vi "Autonomous.vi"() -> ()   [LabVIEW 2023]
doc: "This VI starts when autonomous period begins, and will automatically be terminated when it ends. You can carry out timed or sensor driven operations directly to I/O or to subsystems without needing to return to the caller."
uses:
  <vilib>/Rock Robotics/WPI/Utilities/WPI_GetSetVariantRefNum.vi
  Framework/Robot Global Data.vi
  <vilib>/Rock Robotics/Network Tables/NT Read String.vi
  <vilib>/Rock Robotics/Network Tables/NT Read String Array.vi
  <vilib>/Utility/file.llb/Read Delimited Spreadsheet (string).vi
panel:
  in  "Is Blue Alliance?":bool=TRUE
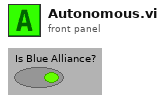
[diagram p1: front panel]
types:
  T1 = typedef "WPI_JoystickDevRef.ctl" = cluster{"Device":T2}
  T2 = typedef "WPI_JoystickDeviceEnum.ctl" = enum16{"USB 0", "USB 1", "USB 2", "USB 3", "USB 4", "USB 5"}
  T3 = typedef "Robot Velocities.ctl" = cluster{"X Velocity":dbl, "Y Velocity":dbl, "Rotational \nVelocity":dbl}
  T4 = typedef "Single Cmd Info.ctl" = cluster{"Name":string, "CPTM.DataType":variant, "All Control Values Variant":cluster{"Name":string, "Variant Data":variant}[], "icon full":T5, "icon scaled":T5, "Path":path, "Subsystem Color":u32}
  T5 = typedef "imagedata.ctl" = cluster{"image type":i32, "image depth":i32, "image":u8[], "mask":u8[], "colors":u32[], "Rectangle":cluster{"left":i16, "top":i16, "right":i16, "bottom":i16}}
  T6 = cluster{"Name":string, "vi reference":refnum<vi>, i32[], variant[]}
  T7 = cluster{dbl, "Command out":cluster{"Name":string, "vi reference":refnum<vi>, i32[], variant[]}}
  T8 = cluster{dbl, "Command out":cluster{"Name":string, "vi reference":refnum<vi>, i32[], variant[]}}[]
  T9 = cluster{"Velocities":T3[], "Positions":cluster{"x":dbl, "y":dbl, "th":dbl}[], cluster{dbl, "Command out":cluster{"Name":string, "vi reference":refnum<vi>, i32[], variant[]}}[], "Zero Velocity?":bool[]}
  T10 = typedef "CTRE_PigeonIMU_DeviceRef.ctl" = cluster{"DeviceStatus":errorcluster, "Device Number":u8, "Type":T11, "Device ID":u32, "Handle":u64, "UsageFrame":u32, "Library Path":path}
  T11 = typedef "CTRE_PigeonIMU_ConnectionType.ctl" = u32
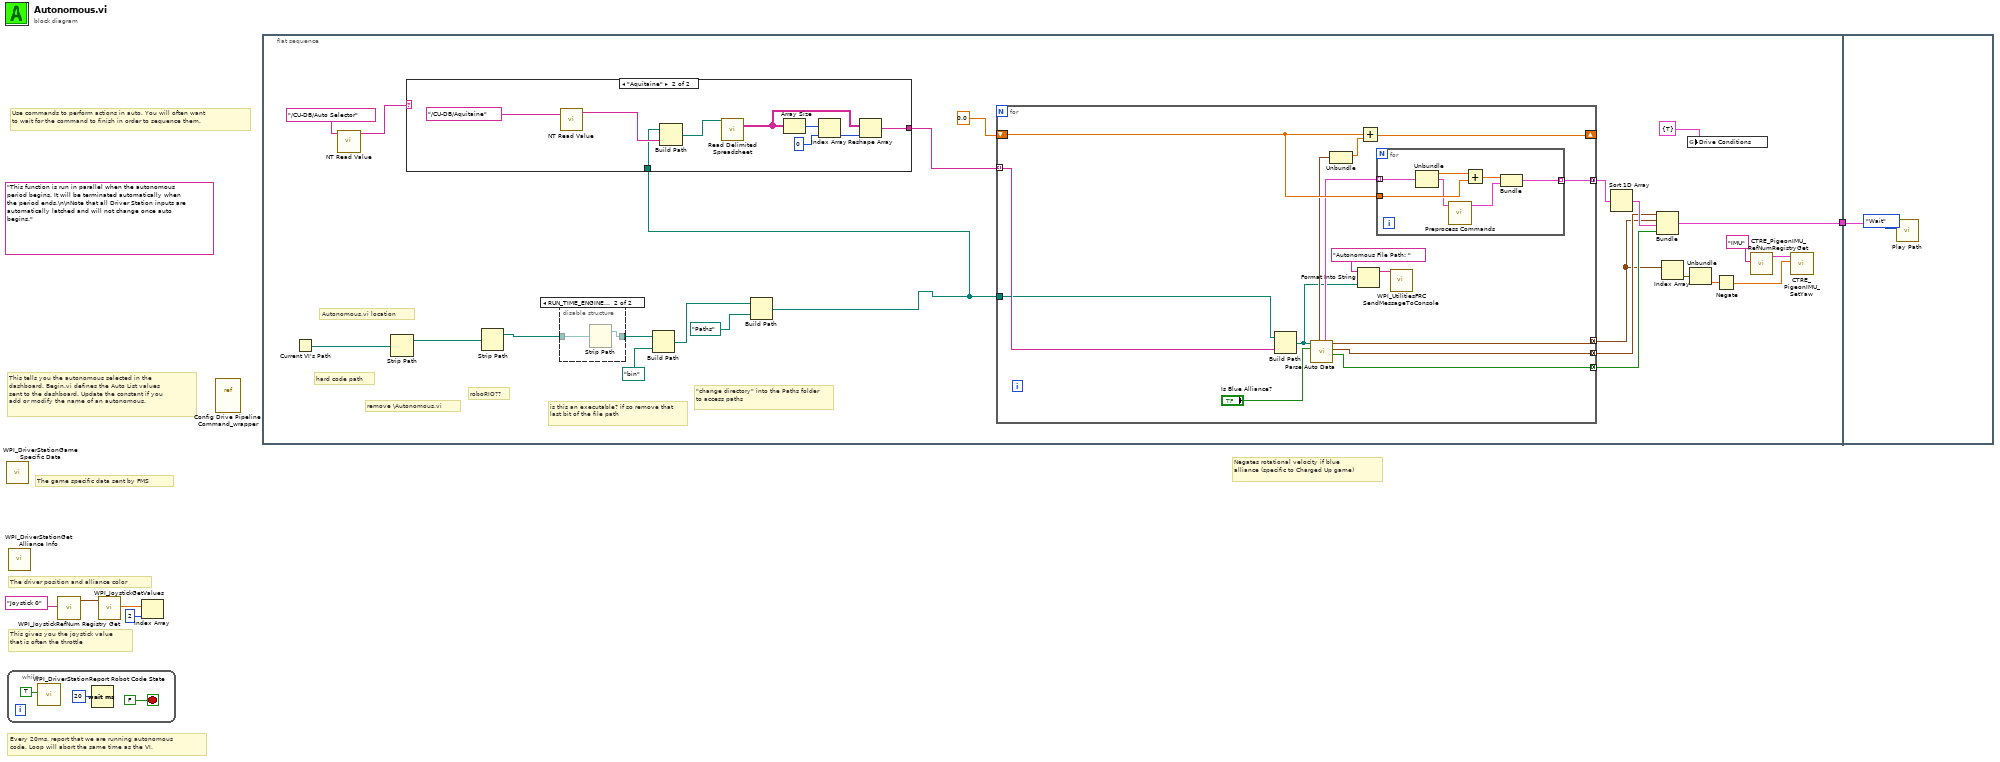
[diagram p0: block diagram]
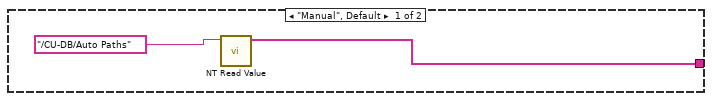
[diagram p3: hidden frame]
diagram:
  (unwired) "This function is run in parallel when the autonomous period begins. It will be terminated automatically when the period ends.\n\nNote that all Driver Station inputs are automatically latched and will not change once auto begins."
  # "Negates rotational velocity if blue alliance (specific to Charged Up game)"
  # "The game specific data sent by FMS"
  # "This tells you the autonomous selected in the \ndashboard. Begin.vi defines the Auto List values\nsent to the dashboard. Update the constant if you\nadd or modify the name of an autonomous."
  # "Every 20ms, report that we are running autonomous\ncode. Loop will abort the same time as the VI."
  # "This gives you the joystick value\nthat is often the throttle"
  # "Use commands to perform actions in auto. You will often want\nto wait for the command to finish in order to sequence them."
  # "The driver position and alliance color"
  n1 = call <vilib>:"WPI_DriverStationGame Specific Data.vi"() -> ()  [unwired: 11 in, 1 out]
  n2 = while {
    stop <- FALSE stop-if-true
    n3 = call <vilib>:"WPI_DriverStationReport Robot Code State.vi"("Autonomous"=TRUE) -> ()  [unwired: 10 in, 1 out]
    n4 = Wait (ms)(milliseconds to wait=u32 20) -> ()  [unwired: 1 out]
  }
  n5 = call <vilib>:"WPI_DriverStationGet Alliance Info.vi"() -> ()  [unwired: 12 out]
  n6 = call <vilib>:"WPI_JoystickRefNum Registry Get.vi"("refnum name"="Joystick 0") -> ("JoystickDevRef"=w4:T1)  [unwired: 1 in, 9 out]
  n7 = call <vilib>:"WPI_JoystickGetValues.vi"("JoystickDevRef"=w4) -> ("Axes"=w3:dbl[])  [unwired: 6 in, 4 out]
  n8 = Index Array(array=w3, index=2) -> ()  [unwired: 1 out]
  n9 = vi-ref "Config Drive Pipeline Command_wrapper.vi"() -> ()  [unwired: 1 out]
  n10 = flat-sequence {
    tunnel: [w23] -> w1
    tunnel: w1 -> [w69]
    frame #0 {
      # "\"change directory\" into the Paths folder to access paths"
      # "is this an executable? if so remove that last bit of the file path"
      # "roboRIO??"
      # "remove \\Autonomous.vi"
      # "Autonomous.vi location"
      # "hard code path"
      n11 = Current VI's Path() -> (path=w16:path)
      n12 = call-poly <vilib>:"NT Read Value.vi"("name"="/CU-DB/Auto Selector") -> ("value"=w12:string)  [unwired: 8 in, 2 out]
      n13 = Strip Path(path=w16) -> (stripped path=w17:path)  [unwired: 1 out]
      n14 = Strip Path(path=w17) -> (stripped path=w19:path)  [unwired: 1 out]
      n15 = disable-structure shown="RUN_TIME_ENGINE==True, Default" {
        disable-tunnel: [w33 w34] -> w18
        disable-tunnel: w19 -> [w33 w35]
        frame condition #0 (active) {
        }
        frame condition #1 {
          n16 = Strip Path(path=w35) -> (stripped path=w34:path)  [unwired: 1 out]
        }
      }
      n17 = Build Path(base path=w18, name or relative path=path "bin") -> (appended path=w10:path)
      n18 = Build Path(base path=w10, name or relative path=path "Paths") -> (appended path=w9:path)
      n19 = case shown="\"Aquitaine\"" w12 {
        tunnel: w9 -> [_ w66]
        tunnel: [w58 w60] -> w13
        frame "Manual", Default {
          n20 = call-poly <vilib>:"NT Read Value.vi"("name"="/CU-DB/Auto Paths") -> ("value"=w58:string[])  [unwired: 8 in, 2 out]
        }
        frame "Aquitaine" {
          n21 = call-poly <vilib>:"NT Read Value.vi"("name"="/CU-DB/Aquitaine") -> ("value"=w67:string)  [unwired: 8 in, 2 out]
          n22 = Build Path(base path=w66, name or relative path=w67) -> (appended path=w65:path)
          n23 = call-poly <vilib>:"Read Delimited Spreadsheet.vi"("file path (dialog if empty)"=w65) -> ("all rows"=w61:string[][])  [unwired: 9 in, 5 out]
          n24 = Array Size(array=w61) -> (size(s)=w64:i32[])
          n25 = Index Array(array=w64, index=0) -> (element=w62:i32)
          n26 = Reshape Array(w61, w62) -> (w60:string[])
        }
      }
      n27 = for {
        tunnel: [w44] -> w22 mode=concatenating
        tunnel: [w45] -> w21 mode=concatenating
        shift-right: [w50] -> _
        shift-left: 0.0 -> [w48]
        tunnel: [w49] -> w29 mode=concatenating
        tunnel: [w42] -> w24 mode=concatenating
        tunnel: w9 -> [w37]
        tunnel: w13 -> [w38] mode=indexing
        n28 = Build Path(base path=w37, name or relative path=w38) -> (appended path=w41:path)
        n29 = call "Parse Auto Data.vi"("Is Blue Alliance?"="Is Blue Alliance?", "path"=w41) -> ("Zero Velocity?"=w42:bool[], "Velocities"=w44:T3[], "Positions"=w45:cluster{"x":dbl, "y":dbl, "th":dbl}[], "Commands out"=w43:cluster{"Time (s)":dbl, T4, bool}[], "Overall"=w47:cluster{"Time (s)":dbl, "Distance (ft)":dbl})  [unwired: 5 in]
        n30 = Unbundle(w47) -> ("Time (s)"=w36:dbl)  [unwired: 1 out]
        n31 = Format Into String(initial string="Autonomous File Path: ", w41) -> (resulting string=w40:string)  [unwired: 2 in, 1 out]
        n32 = Add(x=w48, y=w36) -> (x+y=w50:dbl)
        n33 = for {
          tunnel: w48 -> [w56]
          tunnel: w43 -> [w55] mode=indexing
          tunnel: [w51] -> w49 mode=indexing
          n34 = Unbundle(w55) -> ("Time (s)"=w57:dbl, w54:T4)  [unwired: 1 out]
          n35 = call "Preprocess Commands.vi"("Command In"=w54) -> ("Command out"=w52:T6)  [unwired: 10 in]
          n36 = Add(x=w57, y=w56) -> (x+y=w53:dbl)
          n37 = Bundle(w53, "Command out"=w52) -> (w51:T7)  [unwired: 1 in]
        }
        n38 = call <vilib>:"WPI_UtilitiesFRC SendMessageToConsole.vi"("Message"=w40) -> ()  [unwired: 14 in, 1 out]
      }
      n39 = Sort 1D Array(array=w29) -> (sorted array=w25:T8)
      n40 = Bundle("Velocities"=w22, "Positions"=w21, w25, "Zero Velocity?"=w24) -> (w23:T9)  [unwired: 1 in]
      n41 = Index Array(array=w21) -> (element=w28:cluster{"x":dbl, "y":dbl, "th":dbl})  [unwired: 1 in]
      n42 = global write "Robot Global Data.vi" "Drive Conditions"(cluster{"Field Centric":bool} {"Field Centric"=TRUE} ("Drive Conditions")) -> ()
      n43 = Unbundle(w28) -> ("th"=w27:dbl)  [unwired: 2 out]
      n44 = Negate(x=w27) -> (-x=w26:dbl)
      n45 = call <vilib>:"CTRE_PigeonIMU_RefNumRegistryGet.vi"("refnum name"="IMU") -> ("PigeonIMUDevRef"=w32:T10)  [unwired: 9 in, 1 out]
      n46 = call <vilib>:"CTRE_PigeonIMU_SetYaw.vi"("Value"=w26, "PigeonIMUDevRef"=w32) -> ()  [unwired: 8 in, 2 out]
    }
    frame #1 {
      n47 = call "Play Path.vi"("Synchronization"=enum16{"Start", "Wait"}."Wait", "Auto Data"=w69) -> ()  [unwired: 9 in, 1 out]
    }
  }
